vi "Mark Persisted.vi"(10 "Entity ID":T1, 11 "Entity in":refnum<class "Entity.lvclass">) -> (3 "Entity out":refnum<class "Entity.lvclass">)   [LabVIEW 2022 SP3, in "Conditum.lvlib" / "Entity.lvclass"]
uses:
  Entity.lvclass
  Entity State.ctl
  Conditum.lvlib
  Entity ID.ctl
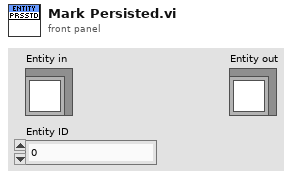
[diagram p1: front panel]
types:
  T1 = typedef "Conditum.lvlib/Entity ID.ctl" = i64
  T2 = typedef "Conditum.lvlib/Entity State.ctl" = enum16{"New", "Managed", "Detached", "Removed"}
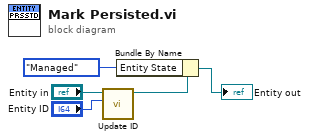
[diagram p0: block diagram]
diagram:
  n1 = call "Update ID.vi"("Entity ID"="Entity ID", "Entity in"="Entity in") -> ("Entity out"=w3:refnum<class "Entity.lvclass">)  [unwired: 9 in]
  n2 = Bundle By Name(cluster=w3, "Entity State"=Entity_State."Managed") -> (→"Entity out":refnum<class "Entity.lvclass">)
